vi "Mac.vi"(8 "error in (no error)":errorcluster, 10 "Font in":string, 11 "Font":refnum<vi>) -> (0 "error out":errorcluster, 2 "Font out":string)   [LabVIEW 2025]
uses:
  <vilib>/LabVIEW Icon API/lv_icon/lv_icon.lvlib
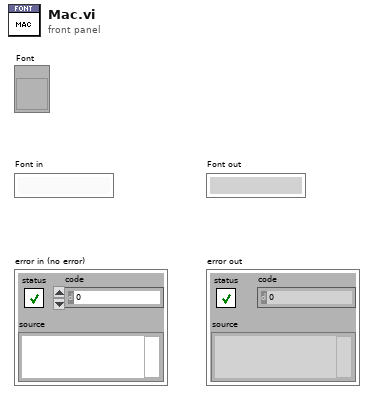
[diagram p1: front panel]
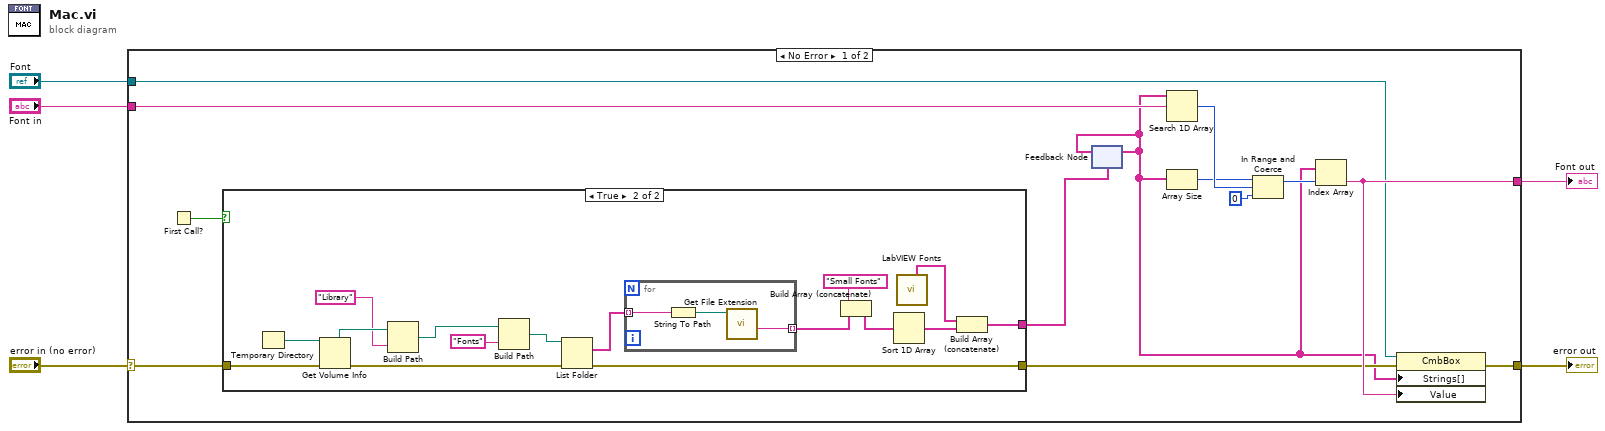
[diagram p0: block diagram]
diagram:
  n1 = case shown="No Error" "error in (no error)" {
    selector: "error in (no error)" -> [w18 w40]
    tunnel: [w17 w40] -> w4
    tunnel: "Font in" -> [w12 w39]
    tunnel: [w11 w39] -> w2
    tunnel: "Font" -> [w10 _]
    frame No Error {
      n2 = First Call?() -> (First Call?: T/F=w8:bool)
      n3 = case shown="True" w8 {
        tunnel: w18 -> [w19 w30]
        tunnel: [_ w25] -> w7
        tunnel: [w19 w23] -> w9
        frame False {
        }
        frame True {
          n4 = Temporary Directory() -> (w35:path)
          n5 = Get Volume Info(8:w30, 11:w35) -> (0:w28:errorcluster, 5:w34:path)  [unwired: 4 out]
          n6 = Build Path(base path=w34, name or relative path="Library") -> (appended path=w31:path)
          n7 = Build Path(base path=w31, name or relative path="Fonts") -> (appended path=w29:path)
          n8 = List Folder(path=w29, error in=w28) -> (filenames=w27:string[], error out=w23:errorcluster)  [unwired: 4 out]
          n9 = for {
            tunnel: w27 -> [w38] mode=indexing
            tunnel: [w36] -> w21 mode=indexing
            n10 = String To Path(string=w38) -> (path=w37:path)
            n11 = call <vilib>:"Get File Extension.vi"("file"=w37) -> ("filename without extension"=w36:string)  [unwired: 1 in, 9 out]
          }
          n12 = Build Array (concatenate)("Small Fonts", w21) -> (w20:string[])
          n13 = Sort 1D Array(array=w20) -> (sorted array=w26:string[])
          n14 = call <vilib>:"LabVIEW Fonts.vi"() -> ("Additional Fonts"=w24:string[])  [unwired: 1 in, 10 out]
          n15 = Build Array (concatenate)(w24, w26) -> (w25:string[])
        }
      }
      n16 = feedback #1(w7) -> (w6:string[])
      n17 = feedback-in #1(w6) -> ()
      n18 = Search 1D Array(1D array=w6, element=w12) -> (index of element=w16:i32)  [unwired: 1 out]
      n19 = Array Size(array=w6) -> (size(s)=w13:i32)
      n20 = In Range and Coerce(upper limit=w13, x=w16, lower limit=0 ("x")) -> (coerced(x)=w14:i32)  [unwired: 1 out]
      n21 = Index Array(array=w6, index=w14) -> (element=w11:string)
      n22 = property class="CmbBox"(reference=w10, error in=w9, "Strings[]"=w6, "Value"=w11) -> (error out=w17:errorcluster)  [unwired: 1 out]
    }
    frame Error {
    }
  }
  "error out" <- w4
  "Font out" <- w2
